vi "Write Config Array.vi"(2 "error in (no error)":errorcluster, 3 "array":dbl[](array[numeric]) format="%.2f", 4 "Key":string, 5 "input cluster":T1 {"MaxLambdaCurrent [A]" format="%.2f"; "LambdaRates [A/min]" format="%.2f"; "MaxNormalCurrent [A]" format="%.2f"; "StabilitySetting [%]" format="%.2f"; "FieldCurrentRatio [T/A]" format="%.2f"; "SwitchWaitTime [s]" format="%.2f"; "SwitchHtrCurrent [mA]" format="%.2f"; "TrainRates [A/min]" format="%.2f"; "NormalRates [A/min]" format="%.2f"; "Breakpts [A]" format="%.2f"}) -> (0 "error out":errorcluster, 1 "message":string=" INSTRUCTIONS:\r\rNormal Use:  When using subVIs that incorporate the error in/error out (or error I/O) structure, place this handler where you want to inform the user of an error, typically at the end of the I/O data path, as the last action of the program.  If the error in error? is ERROR, the handler creates a message describing the error and its source.  If the type of dialog = 1 (default), the message is displayed to the user, who can only acknowedge it.  If the type = 2, the user can acknowledge the message or abort execution; aborting a program with active I/O is not recommended.  If the type = 0, no message is displayed; this is used to process the error programmatically, and the error out cluster elements are wired to individual terminals for that reason.  \r\rOther Use:\n\r\nlocal testing.  To test the error code of a subVI or function that does not have the error I/O structure, you can wire its error code and a source string to the local error code and error source inputs.  If error in error? indicates no error and error code is not equal to 0, the local code and source are substituted for the error in values, and error? is set TRUE (ERROR).")   [LabVIEW 2021]
uses:
  <vilib>/Utility/config.llb/Write Key (String).vi
  <vilib>/Utility/config.llb/NI_LVConfig.lvlib
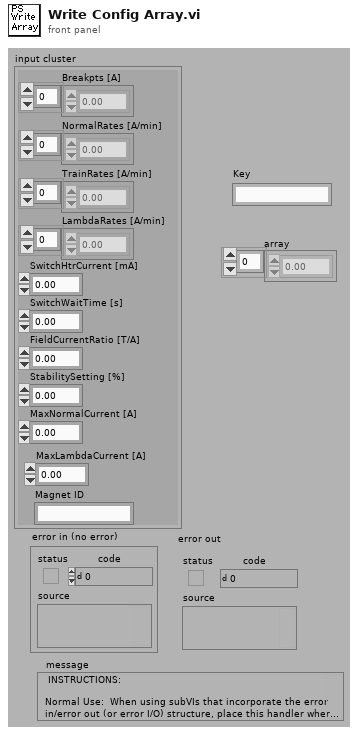
[diagram p1: front panel]
types:
  T1 = cluster{"Breakpts [A]":dbl[], "NormalRates [A/min]":dbl[], "TrainRates [A/min]":dbl[], "SwitchHtrCurrent [mA]":dbl, "SwitchWaitTime [s]":dbl, "FieldCurrentRatio [T/A]":dbl, "StabilitySetting [%]":dbl, "MaxNormalCurrent [A]":dbl, "Magnet ID":string, "LambdaRates [A/min]":dbl[], "MaxLambdaCurrent [A]":dbl}
  T2 = typedef "NI_LVConfig.lvlib/Config Data RefNum.ctl" = refnum<k1>
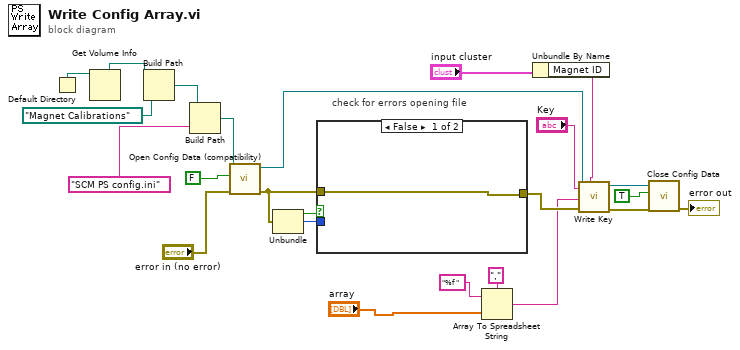
[diagram p0: block diagram]
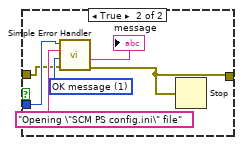
[diagram p2: hidden frame]
diagram:
  # "check for errors opening file"
  n1 = Default Directory() -> (w20:path)
  n2 = Get Volume Info(11:w20) -> (5:w18:path)  [unwired: 1 in, 5 out]
  n3 = Build Path(base path=w18, name or relative path=path "Magnet Calibrations") -> (appended path=w21:path)
  n4 = Build Path(base path=w21, name or relative path="SCM PS config.ini") -> (appended path=w14:path)
  n5 = call <vilib>:"Open Config Data (compatibility).vi"("error in (no error)"="error in (no error)", "create file if necessary (T)"=FALSE ("create file if necessary? (T)"), "configuration file path"=w14) -> ("error out"=w15:errorcluster, "refnum"=w12:T2)  [unwired: 6 in, 1 out]
  n6 = Unbundle(w15) -> ("status"=w17:bool, "code"=w16:i32)  [unwired: 1 out]
  n7 = case shown="False" w17 {
    tunnel: w16 -> [_ w31]
    tunnel: w15 -> [w25 w27]
    tunnel: [w25 w26] -> w13
    frame False {
    }
    frame True {
      w28 = u16 1 items=["no dialog", "OK message", "continue or stop message"] ("type of dialog (OK msg:1)")
      n8 = call <vilib>:"Simple Error Handler.vi"("error code (no error:0)"=w31, "error source (\" \")"="Opening \"SCM PS config.ini\" file" ("error source (\" \")"), "type of dialog (OK msg:1)"=w28, "error in (no error)"=w27) -> ("source out"=→"message":string, "error out"=w26:errorcluster)  [unwired: 1 in, 3 out]
      n9 = Stop(stop? (T)=w26) -> ()
    }
  }
  n10 = Array To Spreadsheet String(delimiter (Tab)=",", array="array", 3:"%f " ("format string")) -> (spreadsheet string=w2:string)
  n11 = Unbundle By Name("input cluster") -> ("Magnet ID"=w5:string)
  n12 = call-poly <vilib>:"Write Key.vi"("section"=w5, "error in (no error)"=w13, "value"=w2, "key"="Key", "refnum"=w12) -> ("error out"=w10:errorcluster, "refnum out"=w9:T2)  [unwired: 4 in, 1 out]
  n13 = call <vilib>:"Close Config Data.vi"("error in (no error)"=w10, "write file if changed (T)"=TRUE ("write configuration file? (F)"), "refnum"=w9) -> ("error out"=→"error out":errorcluster)  [unwired: 7 in, 1 out]
